vi "file test.vi"() -> ()   [LabVIEW 2020]
panel:
  out "error out":errorcluster
  in  "experiment name":string="01_90_01"
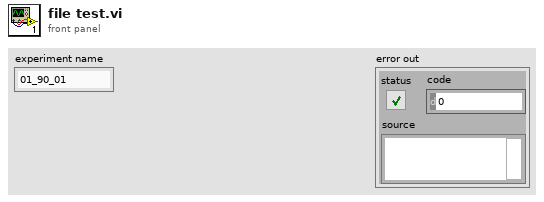
[diagram p1: front panel]
types:
  T1 = enum16{"open", "replace", "create", "open or create", "replace or create", "replace or create with confirmation"}
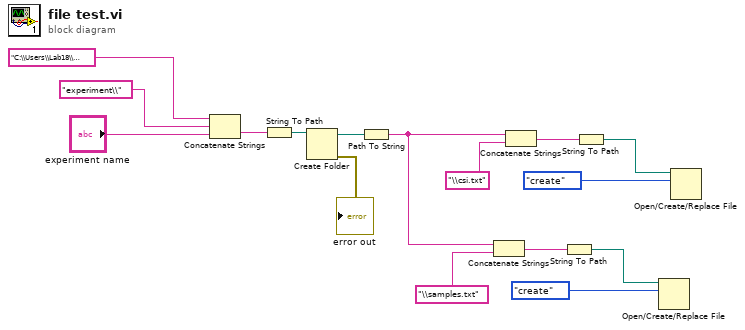
[diagram p0: block diagram]
diagram:
  n1 = Concatenate Strings("C:\\Users\\Lab18\\Documents\\LabVIEW Data\\4-х каналка\\", "experiment\\", "experiment name") -> (w11:string)
  n2 = String To Path(string=w11) -> (path=w10:path)
  n3 = Create Folder(path (use dialog)=w10) -> (created path=w9:path, error out=→"error out":errorcluster)  [unwired: 2 in, 1 out]
  n4 = Path To String(path=w9) -> (string=w2:string)
  n5 = Concatenate Strings(w2, "\\samples.txt") -> (w3:string)
  n6 = Concatenate Strings(w2, "\\csi.txt") -> (w7:string)
  n7 = String To Path(string=w3) -> (path=w5:path)
  n8 = String To Path(string=w7) -> (path=w12:path)
  n9 = Open/Create/Replace File(file path (use dialog)=w5, operation (0:open)=T1."create") -> ()  [unwired: 4 in, 3 out]
  n10 = Open/Create/Replace File(file path (use dialog)=w12, operation (0:open)=T1."create") -> ()  [unwired: 4 in, 3 out]
